vi "GetMotorInfo.vi"(11 "Properties":T2[](array[typedef])) -> (3 "Motor Info":T1)   [LabVIEW 2017, in "McsaStartupAnalysis.lvlib"]
uses:
  <vilib>/addons/InsightCM/Devices/Shared/Mcsa/McsaStartupAnalysis/McsaStartupAnalysis.lvlib
  <vilib>/addons/InsightCM/MessageBus/Base/controls/KeyValuePair.ctl
  <vilib>/addons/InsightCM/Devices/Shared/Mcsa/McsaStartupAnalysis/controls/MotorInfo.ctl
  <vilib>/addons/InsightCM/Utilities/PropertyHelpers/PropertyHelpers.lvlib
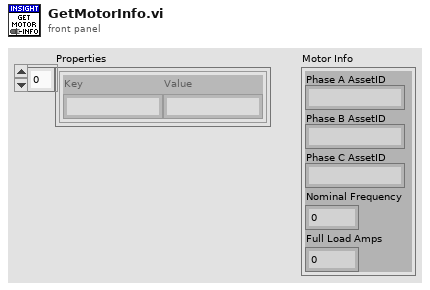
[diagram p1: front panel]
types:
  T1 = typedef "McsaStartupAnalysis.lvlib/MotorInfo.ctl" = cluster{"Phase A AssetID":string, "Phase B AssetID":string, "Phase C AssetID":string, "Nominal Frequency":dbl, "Full Load Amps":dbl}
  T2 = typedef "KeyValuePair.ctl" = cluster{"Key":string, "Value":string}
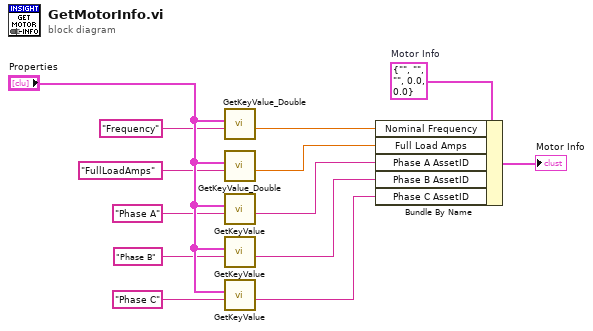
[diagram p0: block diagram]
diagram:
  w5 = T1 {"Phase A AssetID"="", "Phase B AssetID"="", "Phase C AssetID"="", "Nominal Frequency"=0.0, "Full Load Amps"=0.0}  # Motor Info
  n1 = call <vilib>:"GetKeyValue_Double.vi"("key"="Frequency" ("name"), "key value pairs"="Properties") -> ("value"=w13:dbl)  [unwired: 7 in, 2 out]
  n2 = call <vilib>:"GetKeyValue_Double.vi"("key"="FullLoadAmps" ("name"), "key value pairs"="Properties") -> ("value"=w10:dbl)  [unwired: 7 in, 2 out]
  n3 = call <vilib>:"GetKeyValue.vi"("key"="Phase A" ("Name"), "key value pairs"="Properties") -> ("value"=w7:string)  [unwired: 7 in, 2 out]
  n4 = call <vilib>:"GetKeyValue.vi"("key"="Phase B" ("Name"), "key value pairs"="Properties") -> ("value"=w8:string)  [unwired: 7 in, 2 out]
  n5 = call <vilib>:"GetKeyValue.vi"("key"="Phase C" ("Name"), "key value pairs"="Properties") -> ("value"=w9:string)  [unwired: 7 in, 2 out]
  n6 = Bundle By Name(cluster=w5, "Nominal Frequency"=w13, "Full Load Amps"=w10, "Phase A AssetID"=w7, "Phase B AssetID"=w8, "Phase C AssetID"=w9) -> (→"Motor Info":T1)
